vi "Configure AC.vi"(0 "VISA resource name":refnum<visa-resource-name>, 1 "Scan List (Empty)":string, 5 "AC Bandwidth (30)":dbl=30.0, 11 "error in (no error)":errorcluster) -> (4 "VISA resource name out":refnum<visa-resource-name>, 15 "error out":errorcluster)   [LabVIEW 2020, in "Keithley 27XX.lvlib"]
doc: "This VI configures the bandwidth for AC Measurement modes.\n\nBandwidth specifies the lowest frequency of interest for AC measurements.\n\nNote: \n(1) Configure Measurement.vi must be called <B>before</B> configuring the Bandwidth.\n\n(2) This VI will only work when in AC Voltage or AC Current Measurement modes.\n\n(3) The RATE setting determins the bandwidth setting:\nWhen the Slow bandwidth (3Hz to 300kHz) is chosen, the signal goes through an analog RMS converter. The output of the RMS converter goes to a fast (1kHz) sampling A/D and the RMS value is calulated from 1200 digitized samples (1.2s).\nWhen the Medium bandwidth (30Hz to 300kHz) is chosen, the same circuit is used. However, only 120 samples (120ms) are needed for an accurate calculation because the analog RMS converter has turned most of the signal to DC.\nInthe Fast Bandwidth (300Hz to 300kHz), the output of the analog RMS converter (nearly pure DC at these frequencies) is simply measured at 1PLC (16.6ms). The integration rate can be set in the Configure Timing.vi"
uses:
  <instrlib>/Keithley 27XX/Keithley 27XX.lvlib
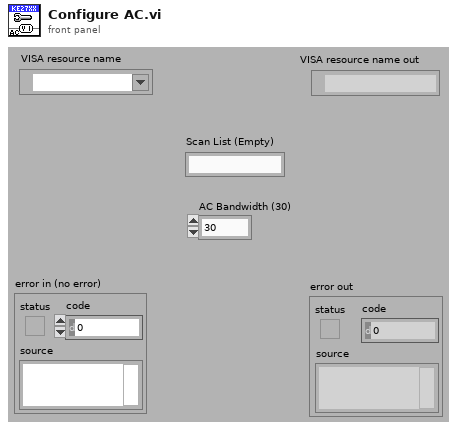
[diagram p1: front panel]
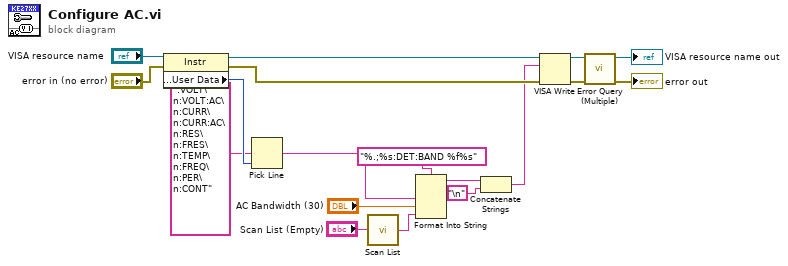
[diagram p0: block diagram]
diagram:
  n1 = property on="Property Node" class="Instr"(reference="VISA resource name", error in="error in (no error)") -> (reference out=w14:refnum<visa-resource-name>, error out=w13:errorcluster, "General Settings:User Data"=w18:u32)
  n2 = Pick Line(multi-line string=":VOLT\n:VOLT:AC\n:CURR\n:CURR:AC\n:RES\n:FRES\n:TEMP\n:FREQ\n:PER\n:CONT", line index=w18) -> (output string=w10:string)  [unwired: 1 in]
  n3 = call <instrlib>:"Scan List.vi"("Scan List (Empty)"="Scan List (Empty)") -> ("Scan List Out"=w8:string)  [unwired: 14 in]
  n4 = Format Into String(format string="%.;%s:DET:BAND %f%s", w10, "AC Bandwidth (30)", w8) -> (resulting string=w1:string)  [unwired: 2 in, 1 out]
  n5 = Concatenate Strings(w1, "\n") -> (w2:string)
  n6 = VISA Write(VISA resource name=w14, write buffer=w2, error in (no error)=w13) -> (VISA resource name out=w7:refnum<visa-resource-name>, error out=w6:errorcluster)  [unwired: 1 out]
  n7 = call <instrlib>:"Error Query (Multiple).vi"("VISA resource name"=w7, "error in (no error)"=w6) -> ("VISA resource name out"=→"VISA resource name out":refnum<visa-resource-name>, "error out"=→"error out":errorcluster)  [unwired: 10 in, 2 out]
